vi "Init.vi"(8 "error in":errorcluster, 10 "<JSON> Const Action Data":string, 11 "Perform Action on Const Channel Strategy in":refnum<class "Perform Action on N Const Channels Strategy.lvclass">) -> (0 "error out":errorcluster, 3 "Perform Action on Const Channel Strategy out":refnum<class "Perform Action on N Const Channels Strategy.lvclass">)   [LabVIEW 2024, in "HAL.lvlib" / "Perform Action on N Const Channels Strategy.lvclass"]
uses:
  Perform Action on N Const Channels Strategy.lvclass
  Perform Action on N Const Channels Strategy.lvclass/Perform Action on N Const Channels Strategy.ctl
  ea423674-1e7e-4dcb-be72-43b9e8909865.vi
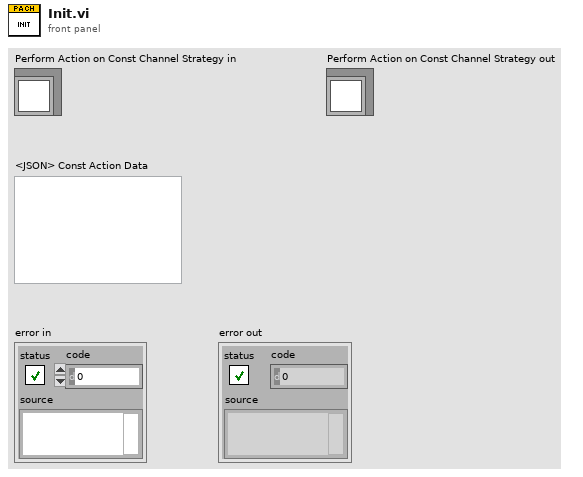
[diagram p1: front panel]
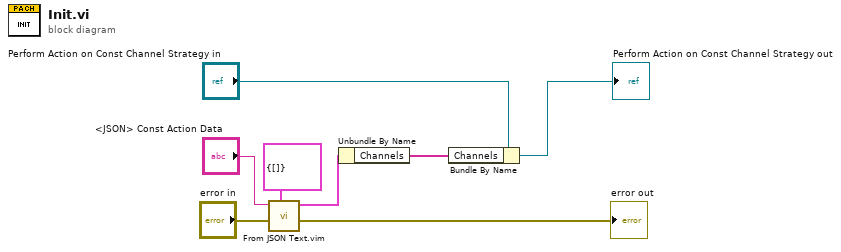
[diagram p0: block diagram]
diagram:
  n1 = call "From JSON Text.vim"("Data Type and Default Value"=cluster{"Channels":string[]} {"Channels"=[]}, "error in (no error)"="error in", "JSON"="<JSON> Const Action Data") -> ("error out"=→"error out":errorcluster, "Data out"=w2:cluster{"Channels":string[]})  [unwired: 7 in]
  n2 = Unbundle By Name(w2) -> ("Channels"=w1:string[])
  n3 = Bundle By Name(cluster="Perform Action on Const Channel Strategy in", "Channels"=w1) -> (→"Perform Action on Const Channel Strategy out":refnum<class "Perform Action on N Const Channels Strategy.lvclass">)
